vi "generate_y_scanner.vi"(8 "error in (no error)":errorcluster, 11 "TrajectoryAK130304ResonanceFlexRIO in":refnum<class "TrajectoryAK130304ResonanceFlexRIO.lvclass">) -> (0 "error out":errorcluster, 3 "TrajectoryAK130304ResonanceFlexRIO out":refnum<class "TrajectoryAK130304ResonanceFlexRIO.lvclass">)   [LabVIEW 2010, in "TrajectoryAK130304ResonanceFlexRIO.lvclass"]
uses:
  TrajectoryAK130304ResonanceFlexRIO.lvclass
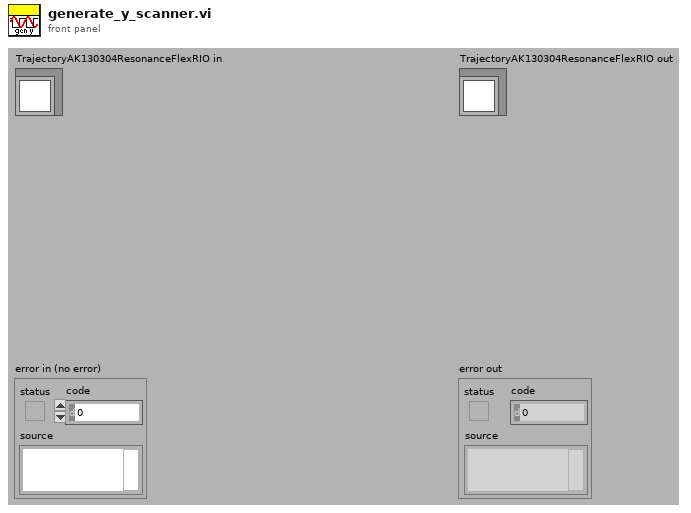
[diagram p1: front panel]
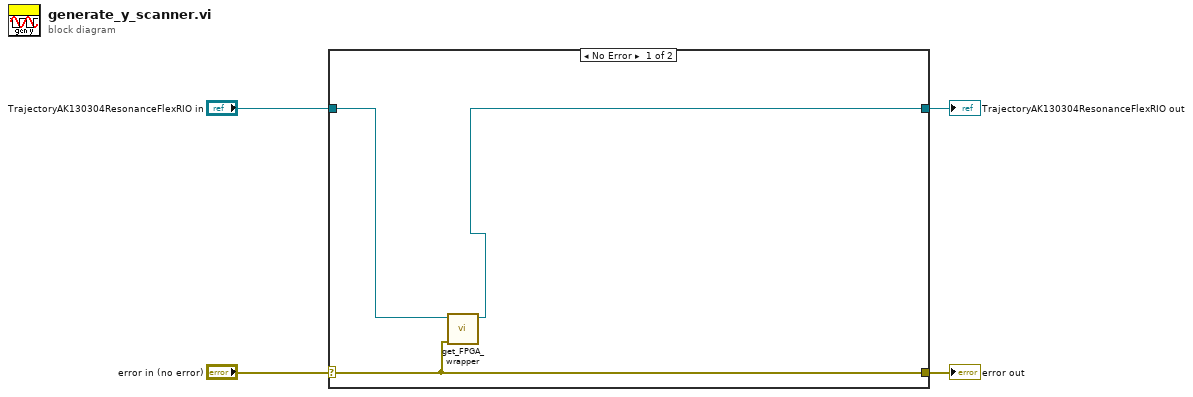
[diagram p0: block diagram]
diagram:
  n1 = case shown="No Error" "error in (no error)" {
    selector: "error in (no error)" -> [w7 w9]
    tunnel: [w7 w9] -> w3
    tunnel: [w5 w8] -> w1
    tunnel: "TrajectoryAK130304ResonanceFlexRIO in" -> [w6 w8]
    frame No Error {
      n2 = call-dynamic "get_FPGA_wrapper.vi"("error in (no error)"=w7, "TrajectoryMG100122GenericFPGA in"=w6) -> ("TrajectoryMG100122GenericFPGA out"=w5:refnum<class "TrajectoryAK130304ResonanceFlexRIO.lvclass">)  [unwired: 7 in, 2 out]
    }
    frame Error {
    }
  }
  "error out" <- w3
  "TrajectoryAK130304ResonanceFlexRIO out" <- w1
